vi "notifier_FGV.vi"(7 "Mode":enum16{"Status", "Add", "Access", "Delete"}(ring), 8 "error in (no error)":errorcluster, 10 "ResponseAddr in":string) -> (0 "error out":errorcluster, 1 "Success?":bool=TRUE, 2 "ResponseAddr out":string, 3 "NotifArray":string[](array[string]))   [LabVIEW 2019, in "MsgQ.lvlib"]
uses:
  MsgQ.lvlib
  mmw_Service/TypeDef/NotifierQ.ctl
  mmw_Service/Service.lvlib
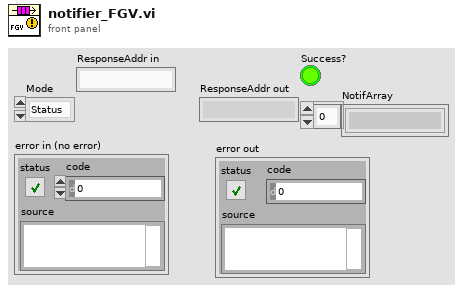
[diagram p1: front panel]
types:
  T1 = typedef "Service.lvlib/NotifierQ.ctl" = cluster{"Data":variant, "Code":dbl}
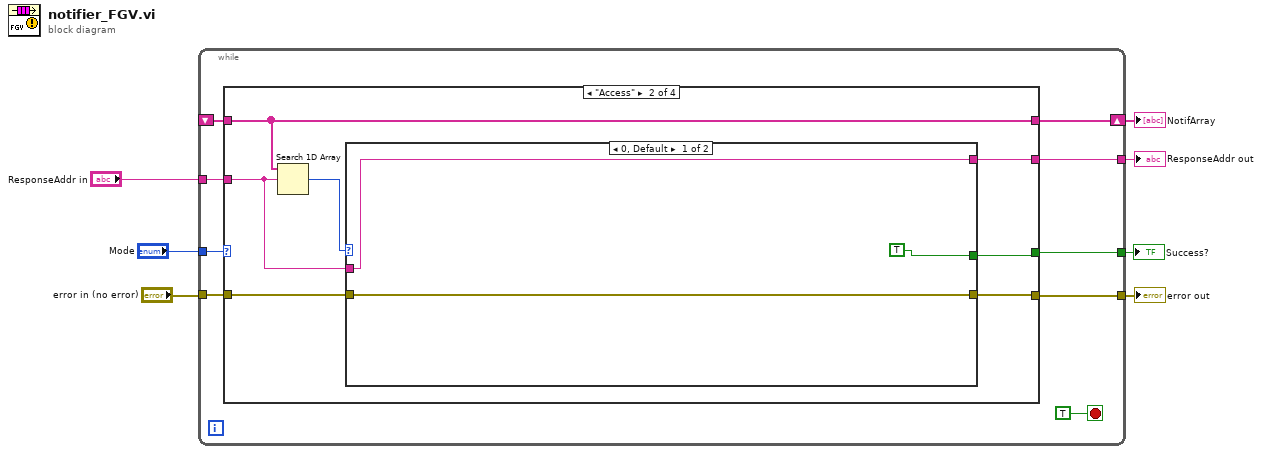
[diagram p0: block diagram]
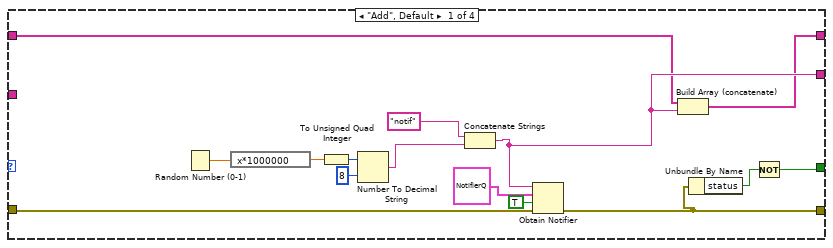
[diagram p2: hidden frame]
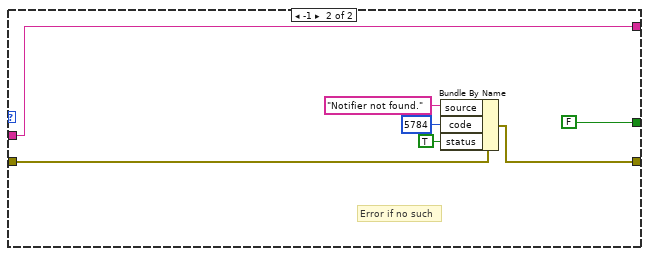
[diagram p3: hidden frame]
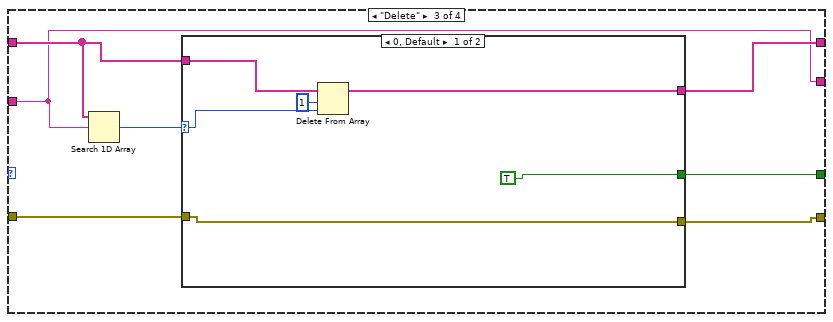
[diagram p4: hidden frame]
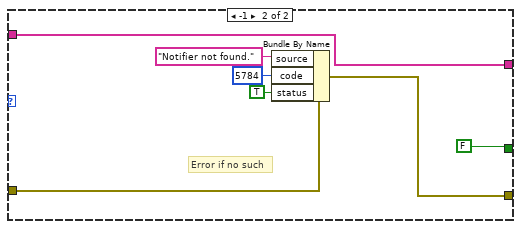
[diagram p5: hidden frame]
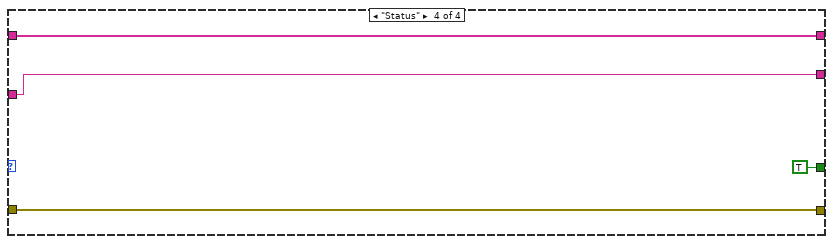
[diagram p6: hidden frame]
diagram:
  n1 = while {
    tunnel: "Mode" -> [w16]
    tunnel: "error in (no error)" -> [w14]
    tunnel: [w13] -> w3
    tunnel: [w12] -> w7
    shift-right: [w11] -> w1
    shift-left: _ -> [w10]
    tunnel: "ResponseAddr in" -> [w9]
    tunnel: [w8] -> w2
    stop <- TRUE stop-if-true
    n2 = case shown="\"Access\"" w16 {
      tunnel: w14 -> [w23 w37 w53 w72]
      tunnel: [w19 w36 w52 w72] -> w13
      tunnel: [w22 w34 w49 w70] -> w12
      tunnel: [w21 w33 w51 w69] -> w11
      tunnel: w10 -> [w20 w33 w55 w69]
      tunnel: w9 -> [_ w35 w49 w70]
      tunnel: [w17 w32 w50 TRUE] -> w8
      frame "Add", Default {
        n3 = Random Number (0-1)() -> (number: 0 to 1=w26:dbl)
        n4 = expression code="x*1000000"(w26) -> (w27:dbl)
        n5 = To Unsigned Quad Integer(1:w27) -> (0:w28:u64)
        n6 = Number To Decimal String(number=w28, width (-)=i16 8) -> (decimal integer string=w31:string)
        n7 = Concatenate Strings("notif" ("name (unnamed)"), w31) -> (w22:string)
        n8 = Obtain Notifier(name (unnamed)=w22, notification data type=T1 {"Data"=variant(enum16{""} enum.""), "Code"=0.0}, create if not found? (T)=TRUE, error in (no error)=w23) -> (error out=w19:errorcluster)  [unwired: 2 out]
        n9 = Build Array (concatenate)(w20, w22) -> (w21:string[])
        n10 = Unbundle By Name(w19) -> ("status"=w18:bool)
        n11 = Not(x=w18) -> (.not. x?=w17:bool)
      }
      frame "Access" {
        n12 = Search 1D Array(1D array=w33, element=w35) -> (index of element=w38:i32)  [unwired: 1 in]
        n13 = case shown="0, Default" w38 {
          tunnel: w37 -> [w39 w48]
          tunnel: [w39 w43] -> w36
          tunnel: w35 -> [w41 w42]
          tunnel: [w41 w42] -> w34
          tunnel: [TRUE FALSE] -> w32
          frame 0, Default {
          }
          frame -1 {
            # "Error if no such"
            n14 = Bundle By Name(cluster=w48, "source"="Notifier not found.", "code"=5784, "status"=TRUE) -> (w43:errorcluster)
          }
        }
      }
      frame "Delete" {
        n15 = Search 1D Array(1D array=w55, element=w49) -> (index of element=w54:i32)  [unwired: 1 in]
        n16 = case shown="0, Default" w54 {
          selector: w54 -> [w60 _]
          tunnel: w55 -> [w61 w62]
          tunnel: w53 -> [w56 w65]
          tunnel: [w56 w64] -> w52
          tunnel: [w58 w62] -> w51
          tunnel: [TRUE FALSE] -> w50
          frame 0, Default {
            n17 = Delete From Array(array=w61, length=1, index=w60) -> (array with subset deleted=w58:string[])  [unwired: 1 out]
          }
          frame -1 {
            # "Error if no such"
            n18 = Bundle By Name(cluster=w65, "source"="Notifier not found.", "code"=5784, "status"=TRUE) -> (w64:errorcluster)
          }
        }
      }
      frame "Status" {
      }
    }
  }
  "ResponseAddr out" <- w7
  "error out" <- w3
  "Success?" <- w2
  "NotifArray" <- w1
